vi "Destroy.vi"(8 "error in (no error)":errorcluster, 11 "MockListImp in":refnum<class "ListImp_RefSpy.lvclass">) -> (0 "error out":errorcluster)   [LabVIEW 2013, in "ListImp_RefSpy.lvclass"]
uses:
  ListImp_RefSpy.lvclass
  source/LapDog.Collections.Lists/ListImp/ListImp.lvclass
  RefnumGlobal.vi
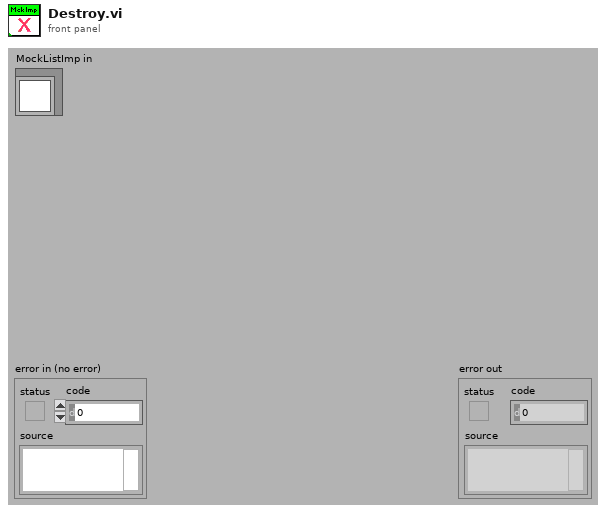
[diagram p1: front panel]
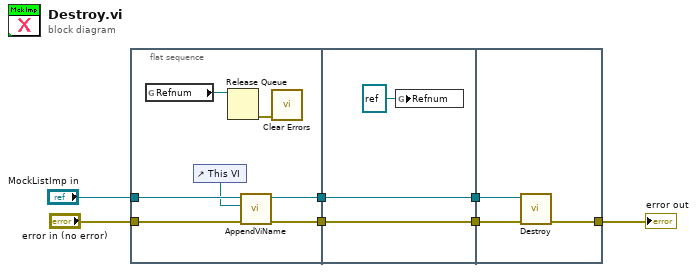
[diagram p0: block diagram]
diagram:
  n1 = flat-sequence {
    tunnel: "MockListImp in" -> [w12]
    tunnel: "error in (no error)" -> [w10]
    tunnel: [w9] -> w2
    tunnel: [w11] -> w1
    tunnel: [w17] -> w4
    tunnel: [w16] -> w3
    tunnel: w2 -> [w17]
    tunnel: w1 -> [w16]
    tunnel: [w20] -> w7
    tunnel: w4 -> [w19]
    tunnel: w3 -> [w18]
    frame #0 {
      n2 = global read "RefnumGlobal.vi" "Refnum"() -> (w14:refnum<queue>)
      n3 = control-ref of="This VI"() -> (w8:refnum<vi>)
      n4 = Release Queue(queue=w14) -> (error out=w13:errorcluster)  [unwired: 2 in, 2 out]
      n5 = call "AppendViName.vi"("error in (no error)"=w10, "VI Refnum"=w8, "MockListImp in"=w12) -> ("error out"=w9:errorcluster, "MockListImp out"=w11:refnum<class "ListImp_RefSpy.lvclass">)  [unwired: 7 in]
      n6 = call <vilib>:"Clear Errors.vi"("error in (no error)"=w13) -> ()  [unwired: 6 in, 1 out]
    }
    frame #1 {
      n7 = global write "RefnumGlobal.vi" "Refnum"(refnum<queue> refnum ("Refnum")) -> ()
    }
    frame #2 {
      n8 = call-parent "Destroy.vi"("error in (no error)"=w19, "ListImp in"=w18) -> ("error out"=w20:errorcluster)  [unwired: 9 in]
    }
  }
  "error out" <- w7
